vi "trigger.vi"(8 "에러 입력":errorcluster, 10 "불리언":bool=TRUE, 11 "FPGA VI 참조 입력":refnum<k20>) -> (0 "에러 출력":errorcluster, 1 "대포발사 Y/N":bool, 2 "불리언 2":bool=TRUE, 3 "FPGA VI 참조 출력":refnum<k20>)   [LabVIEW 2019]
uses:
  global_stop.vi
  <vilib>/Utility/error.llb/Error Cluster From Error Code.vi
  <vilib>/rvi/errors/niLvFpgaAdjustHostInterfaceError.vi
  <vilib>/rvi/interface/nirviReadWriteControl/nirviReadWriteControl.xnode
  <vilib>/rvi/interface/Simulation/niFpgaSimulationCallBeginRW.vi
  NiFpgaLv.dll
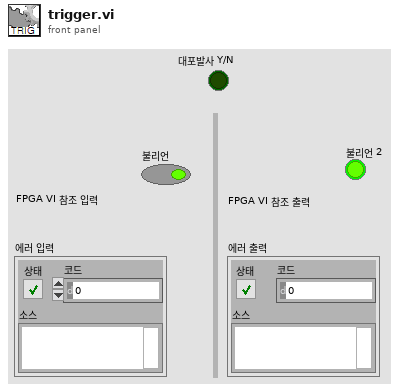
[diagram p1: front panel]
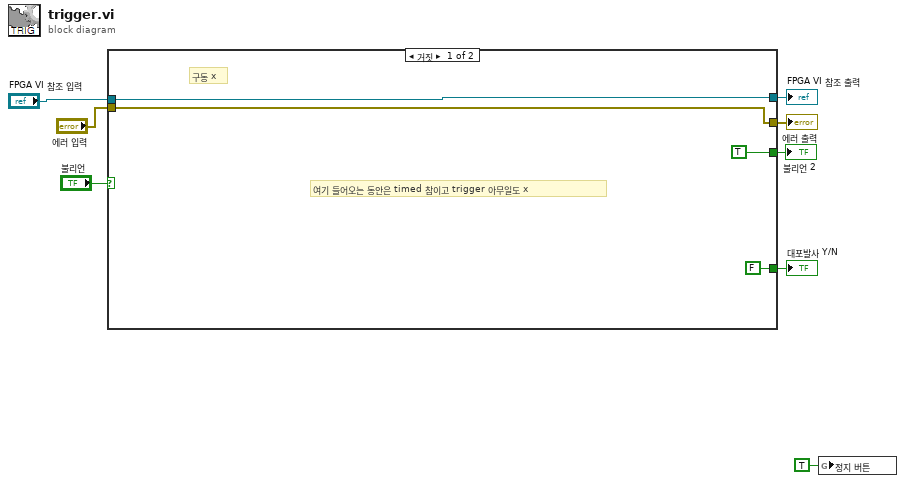
[diagram p0: block diagram]
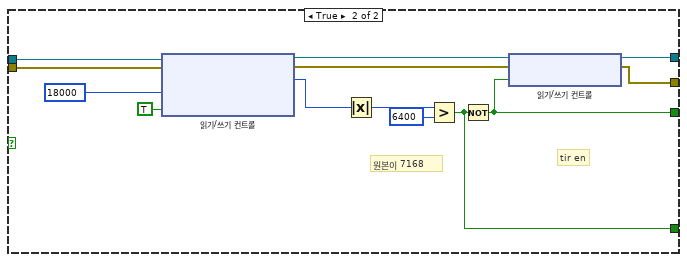
[diagram p2: hidden frame]
diagram:
  n1 = case shown="거짓" "불리언" {
    tunnel: [TRUE w19] -> w7
    tunnel: [FALSE w23] -> w5
    tunnel: [w10 w22] -> w4
    tunnel: [w9 w17] -> w3
    tunnel: "에러 입력" -> [w9 w15]
    tunnel: "FPGA VI 참조 입력" -> [w10 w14]
    frame False {
      # "여기 들어오는 동안은 timed 참이고 trigger 아무일도 x"
      # "구동 x"
    }
    frame True {
      # "tir en"
      # "원본이 7168"
      n2 = xnode "읽기/쓰기 컨트롤"("FPGA VI 참조 입력"=w14, "에러 입력"=w15, "tir_pwm input(escon)"=18000, "tir_DIR"=TRUE) -> ("FPGA VI 참조 출력"=w21:refnum<k20>, "에러 출력"=w20:errorcluster, "tir_Encoder  (4x)"=w16:i32)
      n3 = Absolute Value(x=w16) -> (abs(x)=w24:i32)
      n4 = Greater?(x=w24, y=6400) -> (0:w23:bool)
      n5 = Not(x=w23) -> (.not. x?=w19:bool)
      n6 = xnode "읽기/쓰기 컨트롤"("FPGA VI 참조 입력"=w21, "에러 입력"=w20, "tir_Enable (escon)"=w19) -> ("FPGA VI 참조 출력"=w22:refnum<k20>, "에러 출력"=w17:errorcluster)
    }
  }
  "불리언 2" <- w7
  "대포발사 Y/N" <- w5
  "FPGA VI 참조 출력" <- w4
  "에러 출력" <- w3
  n7 = global write "global_stop.vi" "정지 버튼"(TRUE ("정지 버튼")) -> ()
